vi "dfd_Direct IIR II Transposed Normalization.vi"(7 "scale type":T1, 9 "coefficients b":dbl[](array[numeric]) format="%.2f", 10 "coefficients a":dbl[](array[numeric]) format="%.2f", 11 "x":dbl[](array[numeric])) -> (2 "norm":dbl[](array[numeric]) format="%.2f", 3 "y":dbl[](array[numeric]))   [LabVIEW 2017, in "NI_DigFilter_FXP.lvlib"]
uses:
  <vilib>/addons/Digital Filter Design/NI_DigFilter_FXP.lvlib
  <vilib>/addons/Digital Filter Design/_Objects.llb/DFD Coef Norm Type.ctl
  <vilib>/addons/Digital Filter Design/NI_DigFilterLicensed.lvlib
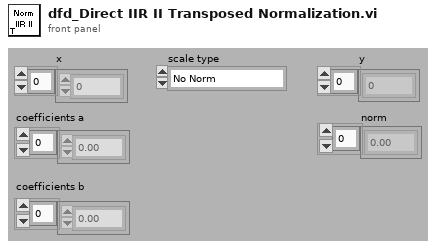
[diagram p1: front panel]
types:
  T1 = typedef "NI_DigFilterLicensed.lvlib/DFD Coef Norm Type.ctl" = enum16{"No Norm", "Time Domain 1-Norm", "Time Domain 2-Norm", "Time Domain Inf-Norm"}
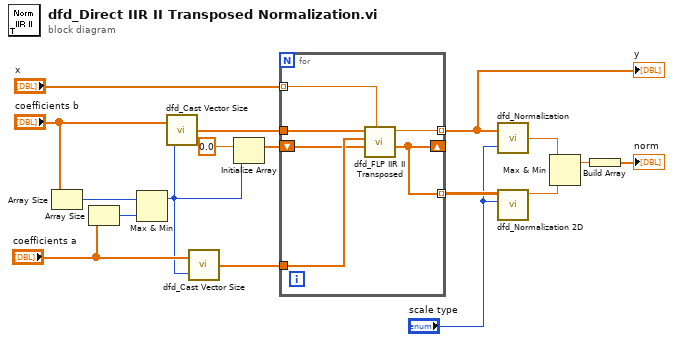
[diagram p0: block diagram]
diagram:
  n1 = Array Size(array="coefficients b") -> (size(s)=w14:i32)
  n2 = Array Size(array="coefficients a") -> (size(s)=w15:i32)
  n3 = Max & Min(x=w14, y=w15) -> (max(x,y)=w10:i32)  [unwired: 1 out]
  n4 = call <vilib>:"dfd_Cast Vector Size.vi"("expected size"=w10, "vector in"="coefficients b") -> ("vector out"=w12:dbl[])
  n5 = call <vilib>:"dfd_Cast Vector Size.vi"("expected size"=w10, "vector in"="coefficients a") -> ("vector out"=w9:dbl[])
  n6 = Initialize Array(0.0 ("element"), w10) -> (w17:dbl[])
  n7 = for {
    shift-right: [w19] -> _
    shift-left: w17 -> [w21]
    tunnel: [w20] -> w6 mode=indexing
    tunnel: w9 -> [w23]
    tunnel: w12 -> [w22]
    tunnel: [w19] -> w7 mode=indexing
    tunnel: "x" -> [w18] mode=indexing
    (unwired) 0.0 ("element")
    n8 = call <vilib>:"dfd_FLP IIR II Transposed.vi"("x"=w18, "states in"=w21, "coefficients a"=w23, "coefficients b"=w22) -> ("states out"=w19:dbl[], "y"=w20:dbl)  [unwired: 6 out]
  }
  "y" <- w6
  n9 = call <vilib>:"dfd_Normalization.vi"("scale type"="scale type", "h(n)"=w6) -> ("norm"=w4:dbl)
  n10 = call <vilib>:"dfd_Normalization 2D.vi"("scale type"="scale type", "2D Array (col-major)"=w7) -> ("max norm"=w3:dbl)  [unwired: 1 in, 8 out]
  n11 = Max & Min(x=w4, y=w3) -> (max(x,y)=w2:dbl)  [unwired: 1 out]
  n12 = Build Array(w2) -> (→"norm":dbl[])
